vi "LEBITVacuum.GetAddress.vi"(2 "channel# (dec)":i32, 3 "base Actual addr. (oct)":string) -> (0 "is a boolean?":bool, 1 "act. addr. (oct)":string)   [LabVIEW 2014, in "LEBITVacuum.lvlib"]
uses:
  LEBITVacuum.lvlib
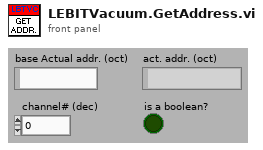
[diagram p1: front panel]
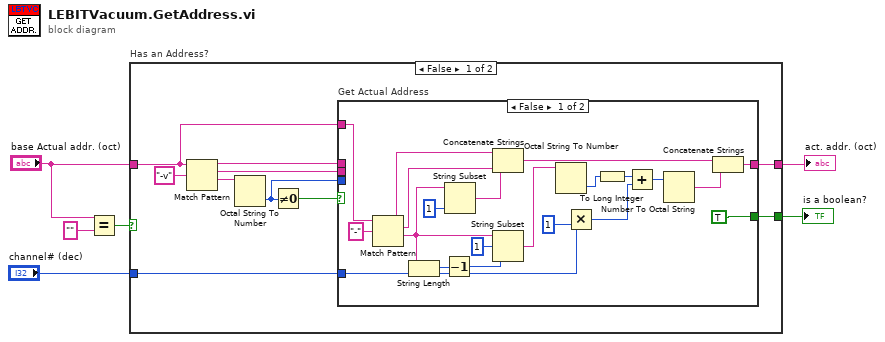
[diagram p0: block diagram]
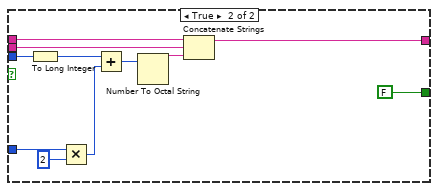
[diagram p2: hidden frame]
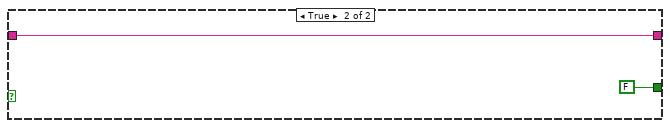
[diagram p3: hidden frame]
diagram:
  n1 = Equal?(x="base Actual addr. (oct)", y="") -> (x = y?=w4:bool)
  n2 = case "Has an Address?" shown="False" w4 {
    tunnel: "channel# (dec)" -> [w16 _]
    tunnel: "base Actual addr. (oct)" -> [w10 w49]
    tunnel: [w9 w49] -> w3
    tunnel: [w8 FALSE] -> w2
    frame False {
      n3 = Match Pattern(string=w10, regular expression="-v" ("search string")) -> (before substring=w12:string, match substring=w11:string, after substring=w14:string)  [unwired: 1 in, 1 out]
      n4 = Octal String To Number(4:w14) -> (0:w13:u32)  [unwired: 2 in, 1 out]
      n5 = Not Equal To 0?(x=w13) -> (x != 0?=w7:bool)
      n6 = case "Get Actual Address" shown="False" w7 {
        tunnel: w16 -> [w36 w46]
        tunnel: w10 -> [w24 _]
        tunnel: [w34 w44] -> w9
        tunnel: w13 -> [_ w39]
        tunnel: w12 -> [_ w43]
        tunnel: w11 -> [_ w42]
        tunnel: [TRUE FALSE] -> w8
        frame False {
          n7 = Match Pattern(string=w24, regular expression="-") -> (before substring=w29:string, match substring=w28:string, after substring=w27:string)  [unwired: 1 in, 1 out]
          n8 = String Length(string=w27) -> (length=w32:i32)
          n9 = Decrement(x=w32) -> (x-1=w30:i32)
          n10 = String Subset(string=w27, length (rest)=1 ("length (rest)")) -> (substring=w25:string)  [unwired: 1 in]
          n11 = Concatenate Strings(w29, w28, w25) -> (w23:string)
          n12 = String Subset(string=w27, offset (0)=1, length (rest)=w30) -> (substring=w22:string)
          n13 = Octal String To Number(4:w22) -> (0:w18:u32)  [unwired: 2 in, 1 out]
          n14 = Multiply(x=w36, y=1) -> (x*y=w20:i32)
          n15 = To Long Integer(number=w18) -> (32bit integer=w19:i32)
          n16 = Add(x=w19, y=w20) -> (x+y=w37:i32)
          n17 = Number To Octal String(2:w37) -> (0:w35:string)  [unwired: 1 in]
          n18 = Concatenate Strings(w23, w35) -> (w34:string)
        }
        frame True {
          n19 = To Long Integer(number=w39) -> (32bit integer=w40:i32)
          n20 = Multiply(x=w46, y=2) -> (x*y=w41:i32)
          n21 = Add(x=w40, y=w41) -> (x+y=w48:i32)
          n22 = Number To Octal String(2:w48) -> (0:w45:string)  [unwired: 1 in]
          n23 = Concatenate Strings(w43, w42, w45) -> (w44:string)
        }
      }
    }
    frame True {
    }
  }
  "act. addr. (oct)" <- w3
  "is a boolean?" <- w2
